vi "Measurement Done.vi"(6 "Array of Hardware":refnum<class "Hardware.lvclass">[](array[class]), 8 "error in (no error)":errorcluster, 9 "Measurement Name":string, 10 "GUID":string, 11 "Controller in":refnum<class "Controller.lvclass">) -> (0 "error out":errorcluster, 3 "Controller out":refnum<class "Controller.lvclass">)   [LabVIEW 2015, in "Controller Actor.lvlib" / "Controller.lvclass"]
uses:
  Controller.lvclass
  Hardware/Hardware.lvclass
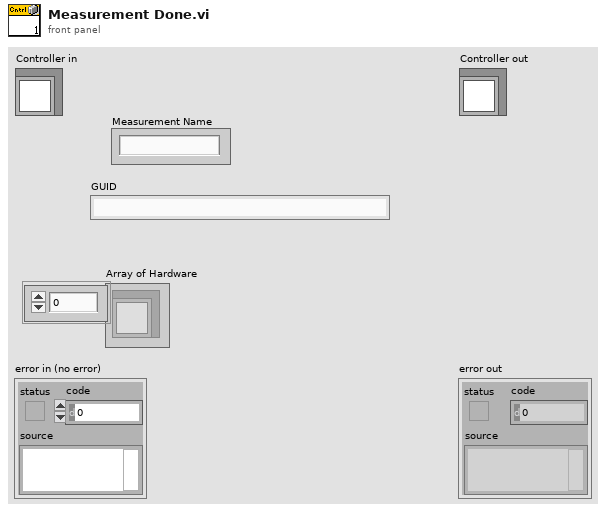
[diagram p1: front panel]
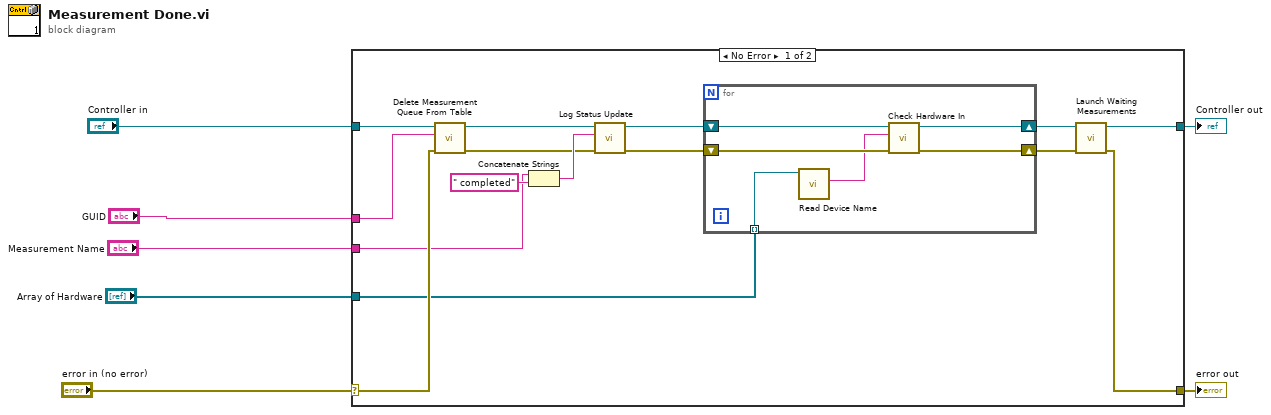
[diagram p0: block diagram]
diagram:
  n1 = case shown="No Error" "error in (no error)" {
    selector: "error in (no error)" -> [w12 w30]
    tunnel: [w11 w30] -> w6
    tunnel: [w21 w29] -> w4
    tunnel: "Controller in" -> [w15 w29]
    tunnel: "GUID" -> [w16 _]
    tunnel: "Measurement Name" -> [w10 _]
    tunnel: "Array of Hardware" -> [w9 _]
    frame No Error {
      n2 = call "Delete Measurement Queue From Table.vi"("error in (no error)"=w12, "Unique Identifier"=w16, "Controller in"=w15) -> ("error out"=w8:errorcluster, "Controller out"=w18:refnum<class "Controller.lvclass">)  [unwired: 7 in]
      n3 = Concatenate Strings(w10, " completed" ("string")) -> (w19:string)
      n4 = call-dynamic "Log Status Update.vi"("error in (no error)"=w8, "String"=w19, "Controller in"=w18) -> ("error out"=w14:errorcluster, "Controller out"=w17:refnum<class "Controller.lvclass">)  [unwired: 7 in]
      n5 = for {
        shift-right: [w27] -> w22
        shift-left: w17 -> [w28]
        shift-right: [w25] -> w13
        shift-left: w14 -> [w26]
        tunnel: w9 -> [w23] mode=indexing
        n6 = call "Read Device Name.vi"("Analog in"=w23) -> ("Device Name"=w24:string)  [unwired: 8 in, 2 out]
        n7 = call "Check Hardware In.vi"("error in (no error)"=w26, "Hardware Name"=w24, "Controller in"=w28) -> ("error out"=w25:errorcluster, "Controller out"=w27:refnum<class "Controller.lvclass">)  [unwired: 7 in]
      }
      n8 = call "Launch Waiting Measurements.vi"("error in (no error)"=w13, "Controller in"=w22) -> ("error out"=w11:errorcluster, "Controller out"=w21:refnum<class "Controller.lvclass">)  [unwired: 8 in]
    }
    frame Error {
    }
  }
  "error out" <- w6
  "Controller out" <- w4
